vi "Configure Measurement (Pulse Width).vi"(5 "Pulse Width Estimate (50E-9)":dbl=5e-08 format="%^#_6g", 7 "Pulse Width Resolution (1E-9s)":dbl=1e-09, 8 "error in (no error)":errorcluster, 9 "Pulse Width Type (0:Positive)":i32(ring) items=["Positive", "Negative"], 10 "Channel (1:Channel 1)":i32(ring)=1 items=["Channel 1"=1, "Channel 2"=2], 11 "VISA resource name":refnum<visa-resource-name>) -> (0 "error out":errorcluster, 3 "VISA resource name out":refnum<visa-resource-name>)   [LabVIEW 2015, in "Template - Counter.lvlib"]
doc: "Configure the settings required for Pulse Width measurements."
uses:
  <instrlib>/_Template - Counter/Template - Counter.lvlib
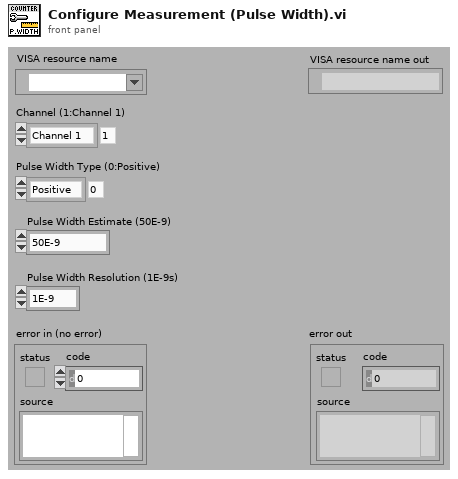
[diagram p1: front panel]
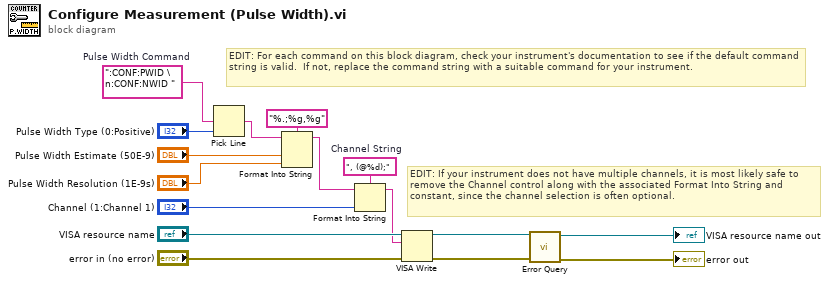
[diagram p0: block diagram]
diagram:
  w3 = ":CONF:PWID \n:CONF:NWID "  # Pulse Width Command
  w12 = ", (@%d);"  # Channel String
  # "EDIT: If your instrument does not have multiple channels, it is most likely safe to remove the Channel control along with the associated Format Into String and constant, since the channel selection is often optional."
  # "EDIT: For each command on this block diagram, check your instrument's documentation to see if the default command string is valid.  If not, replace the command string with a suitable command for your instrument."
  n1 = Pick Line(multi-line string=w3, line index="Pulse Width Type (0:Positive)") -> (output string=w4:string)  [unwired: 1 in]
  n2 = Format Into String(format string="%.;%g,%g", initial string=w4, "Pulse Width Estimate (50E-9)", "Pulse Width Resolution (1E-9s)") -> (resulting string=w5:string)  [unwired: 1 in, 1 out]
  n3 = Format Into String(format string=w12, initial string=w5, "Channel (1:Channel 1)") -> (resulting string=w6:string)  [unwired: 1 in, 1 out]
  n4 = VISA Write(VISA resource name="VISA resource name", write buffer=w6, error in (no error)="error in (no error)") -> (VISA resource name out=w11:refnum<visa-resource-name>, error out=w9:errorcluster)  [unwired: 1 out]
  n5 = call <instrlib>:"Error Query.vi"("error in (no error)"=w9, "VISA resource name"=w11) -> ("error out"=→"error out":errorcluster, "VISA resource name out"=→"VISA resource name out":refnum<visa-resource-name>)  [unwired: 6 in, 2 out]
